vi "Create Message Data Clusters (complex).vi"(8 "error in (no error)":errorcluster, 10 "Message Metadata":T1, 11 "LVClassLibrary in":refnum<vi>) -> (0 "error out":errorcluster, 3 "LVClassLibrary out":refnum<vi>)   [LabVIEW 2019, in "gRPC Scripting Tools.lvlib"]
uses:
  gRPC Scripting Tools.lvlib
  TypeDefs/Message Metadata (Scripting).ctl
  TypeDefs/Message Element Metadata (Scripting).ctl
  TypeDefs/Message Element Type.ctl
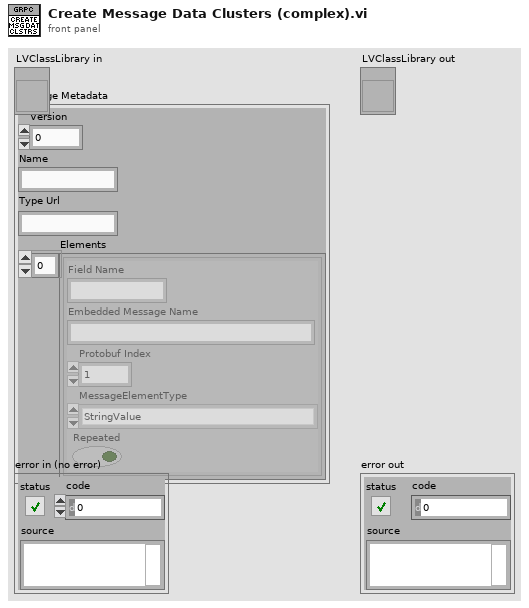
[diagram p1: front panel]
types:
  T1 = typedef "gRPC Scripting Tools.lvlib/Message Metadata (Scripting).ctl" = cluster{"Version":i32, "Name":string, "Type Url":string, "Elements":T2[]}
  T2 = typedef "gRPC Scripting Tools.lvlib/Message Element Metadata (Scripting).ctl" = cluster{"Field Name":string, "Embedded Message Name":string, "Protobuf Index":i32, "MessageElementType":T3, "Repeated":bool}
  T3 = typedef "gRPC Scripting Tools.lvlib/Message Element Type.ctl" = enum32{"Int32Value", "FloatValue", "DoubleValue", "BoolValue", "StringValue", "MessageValue", "Int64Value", "UInt32Value", "UInt64Value", "EnumValue", "Bytes", "Fixed64", "Fixed32", "SFixed64", "SFixed32", "SInt64", "SInt32"}
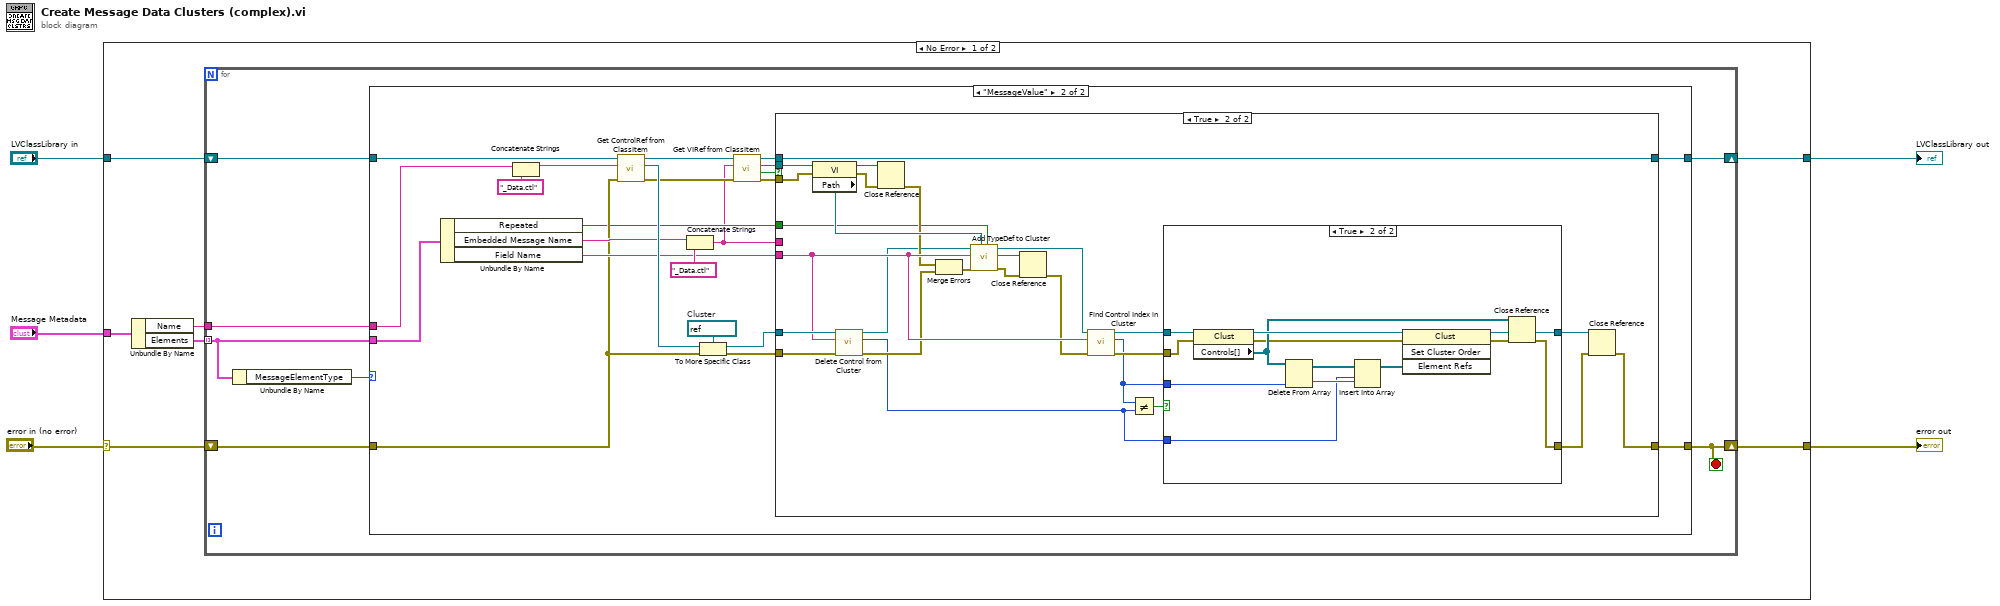
[diagram p0: block diagram]
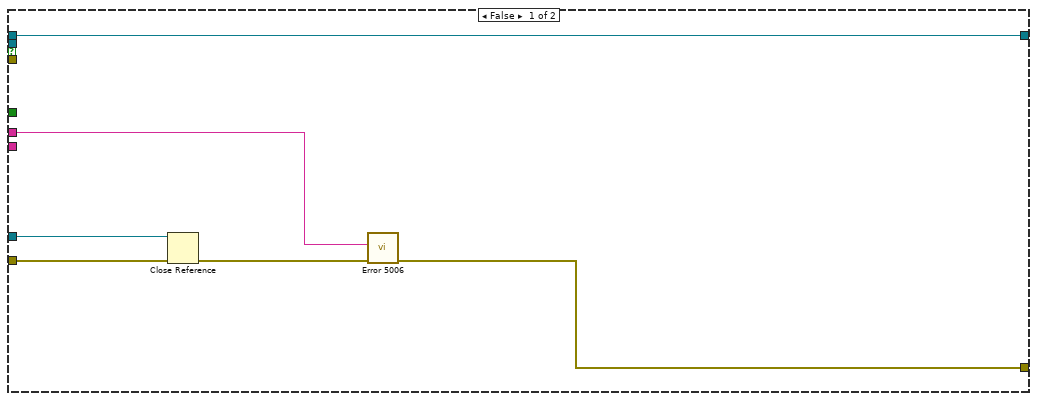
[diagram p3: hidden frame]
diagram:
  n1 = case shown="No Error" "error in (no error)" {
    selector: "error in (no error)" -> [w7 w92]
    tunnel: "Message Metadata" -> [w12 _]
    tunnel: "LVClassLibrary in" -> [w8 w93]
    tunnel: [w9 w92] -> w3
    tunnel: [w10 w93] -> w2
    frame No Error {
      n2 = Unbundle By Name(w12) -> ("Name"=w6:string, "Elements"=w11:T2[])
      n3 = for {
        tunnel: w11 -> [w16] mode=indexing
        shift-right: [w17] -> w10
        shift-left: w8 -> [w18]
        shift-right: [w13] -> w9
        shift-left: w7 -> [w14]
        tunnel: w6 -> [w15]
        stop <- w13 stop-if-true
        n4 = Unbundle By Name(w16) -> ("MessageElementType"=w19:T3)
        n5 = case shown="\"MessageValue\"" w19 {
          tunnel: w16 -> [_ w36]
          tunnel: w18 -> [w21 w41]
          tunnel: [w21 w23] -> w17
          tunnel: w15 -> [_ w40]
          tunnel: w14 -> [w20 w28]
          tunnel: [w20 w34] -> w13
          frame "StringValue", Default {
          }
          frame "MessageValue" {
            w38 = refnum<vi> refnum  # Cluster
            n6 = Unbundle By Name(w36) -> ("Repeated"=w26:bool, "Embedded Message Name"=w35:string, "Field Name"=w29:string)
            n7 = Concatenate Strings(w40, "_Data.ctl" ("string")) -> (w42:string)
            n8 = call "Get ControlRef from ClassItem.vi"("error in (no error)"=w28, "Item Name"=w42, "LVClassLibrary in"=w41) -> ("error out"=w27:errorcluster, "Control ref out"=w39:refnum<vi>, "LVClassLibrary out"=w31:refnum<vi>)  [unwired: 5 in, 1 out]
            n9 = Concatenate Strings(w35, "_Data.ctl" ("string")) -> (w22:string)
            n10 = To More Specific Class(target class=w38, reference=w39, error in=w28) -> (specific class reference=w37:refnum<vi>, error out=w30:errorcluster)
            n11 = call "Get VIRef from ClassItem.vi"("error in (no error)"=w27, "Item Name"=w22, "LVClassLibrary in"=w31) -> ("error out"=w32:errorcluster, "Found ?"=w25:bool, "VIref out"=w33:refnum<vi>, "LVClassLibrary out"=w24:refnum<vi>)  [unwired: 5 in]
            n12 = case shown="True" w25 {
              tunnel: w37 -> [w49 w76]
              tunnel: [w46 w70] -> w34
              tunnel: w33 -> [_ w68]
              tunnel: w32 -> [_ w66]
              tunnel: w30 -> [w48 w65]
              tunnel: w29 -> [_ w64]
              tunnel: w26 -> [_ w52]
              tunnel: w24 -> [w50 w51]
              tunnel: [w50 w51] -> w23
              tunnel: w22 -> [w45 _]
              frame False {
                n13 = Close Reference(reference=w49, error in (no error)=w48) -> (error out=w47:errorcluster)
                n14 = call "Error 5006.vi"("error in (no error)"=w47, "Embedded Message Name"=w45) -> ("error out"=w46:errorcluster)  [unwired: 9 in]
              }
              frame True {
                n15 = property class="VI"(reference=w68, error in=w66) -> (reference out=w62:refnum<vi>, error out=w61:errorcluster, "Path"=w67:path)
                n16 = call "Delete Control from Cluster.vi"("error in (no error)"=w65, "Control Name in"=w64, "Cluster ref in"=w76) -> ("error out"=w63:errorcluster, "Deleted Index"=w53:i32, "Cluster ref out"=w58:refnum<vi>)  [unwired: 6 in]
                n17 = Close Reference(reference=w62, error in (no error)=w61) -> (error out=w60:errorcluster)
                n18 = Merge Errors(w60, w63) -> (w59:errorcluster)
                n19 = call "Add TypeDef to Cluster.vi"("isArray (F)"=w52, "TypeDef path"=w67, "error in (no error)"=w59, "Field Name"=w64, "Owning cluster ref in"=w58) -> ("error out"=w55:errorcluster, "Control ref out"=w56:refnum<vi>, "Owning cluster ref out"=w57:refnum<vi>)  [unwired: 4 in]
                n20 = Close Reference(reference=w56, error in (no error)=w55) -> (error out=w54:errorcluster)
                n21 = call "Find Control Index in Cluster.vi"("error in (no error)"=w54, "Control Name"=w64, "Cluster ref in"=w57) -> ("error out"=w73:errorcluster, "Control Index"=w72:i32, "Cluster ref out"=w74:refnum<vi>)  [unwired: 6 in]
                n22 = Not Equal?(x=w72, y=w53) -> (x != y?=w75:bool)
                n23 = case shown="True" w75 {
                  tunnel: w74 -> [w77 w91]
                  tunnel: w73 -> [w78 w90]
                  tunnel: w72 -> [_ w89]
                  tunnel: w53 -> [_ w86]
                  tunnel: [w78 w81] -> w71
                  tunnel: [w77 w80] -> w69
                  frame False {
                  }
                  frame True {
                    n24 = property class="Clust"(reference=w91, error in=w90) -> (reference out=w85:refnum<vi>, error out=w79:errorcluster, "Controls[]"=w82:refnum<vi>[])
                    n25 = Delete From Array(array=w82, index=w89) -> (deleted portion=w87:refnum<vi>, array with subset deleted=w88:refnum<vi>[])  [unwired: 1 in]
                    n26 = Insert Into Array(array=w88, index=w86, new element=w87) -> (w84:refnum<vi>[])
                    n27 = invoke class="Clust" method="Set Cluster Order"(reference=w85, error in=w79, "Element Refs"=w84) -> (reference out=w80:refnum<vi>, error out=w83:errorcluster)  [unwired: 1 in, 2 out]
                    n28 = Close Reference(reference=w82, error in (no error)=w83) -> (error out=w81:errorcluster)
                  }
                }
                n29 = Close Reference(reference=w69, error in (no error)=w71) -> (error out=w70:errorcluster)
              }
            }
          }
        }
      }
    }
    frame Error {
    }
  }
  "error out" <- w3
  "LVClassLibrary out" <- w2
